vi "GUI_Pico_DMPicos.vi"() -> ()   [LabVIEW 2020]
uses:
  Shared/GUI_Template/GUI_master/tcp_new_data_event.ctl
  Shared/GUI_Template/GUI_master/tcp new data cluster.ctl
panel:
  in  "Position.device 1::2":dbl caption="Position X" min=-10000.0 max=10000.0
  in  "relativeMove.device 5neg::2":bool
  in  "relativeMove.device 5pos::2":bool
  in  "relativeMove.device 4neg::2":bool
  in  "relativeMove.device 4pos::2":bool
  in  "StepSize.device 5::2":dbl caption="StepSize Channel 5" min=0.0 max=1000.0
  in  "StepSize.device 4::2":dbl caption="StepSize Channel 4" min=0.0 max=1000.0
  in  "relativeMove.device 1neg::2":bool
  in  "relativeMove.device 1pos::2":bool
  in  "relativeMove.device 2pos::2":bool
  in  "relativeMove.device 2neg::2":bool
  in  "StepSize.device 2::2":dbl caption="StepSize Y-axis (2)" min=0.0 max=100.0
  in  "StepSize.device 1::2":dbl caption="StepSize X-axis (1)" min=0.0 max=100.0
  in  "GUIdevice 2":string="MCD-LT-PicoBooster"
  in  "stop":bool
  out "tcp data event":T1
  out "error IO 2":errorcluster
  # "XPW Input"
  # "PreAmp Input"
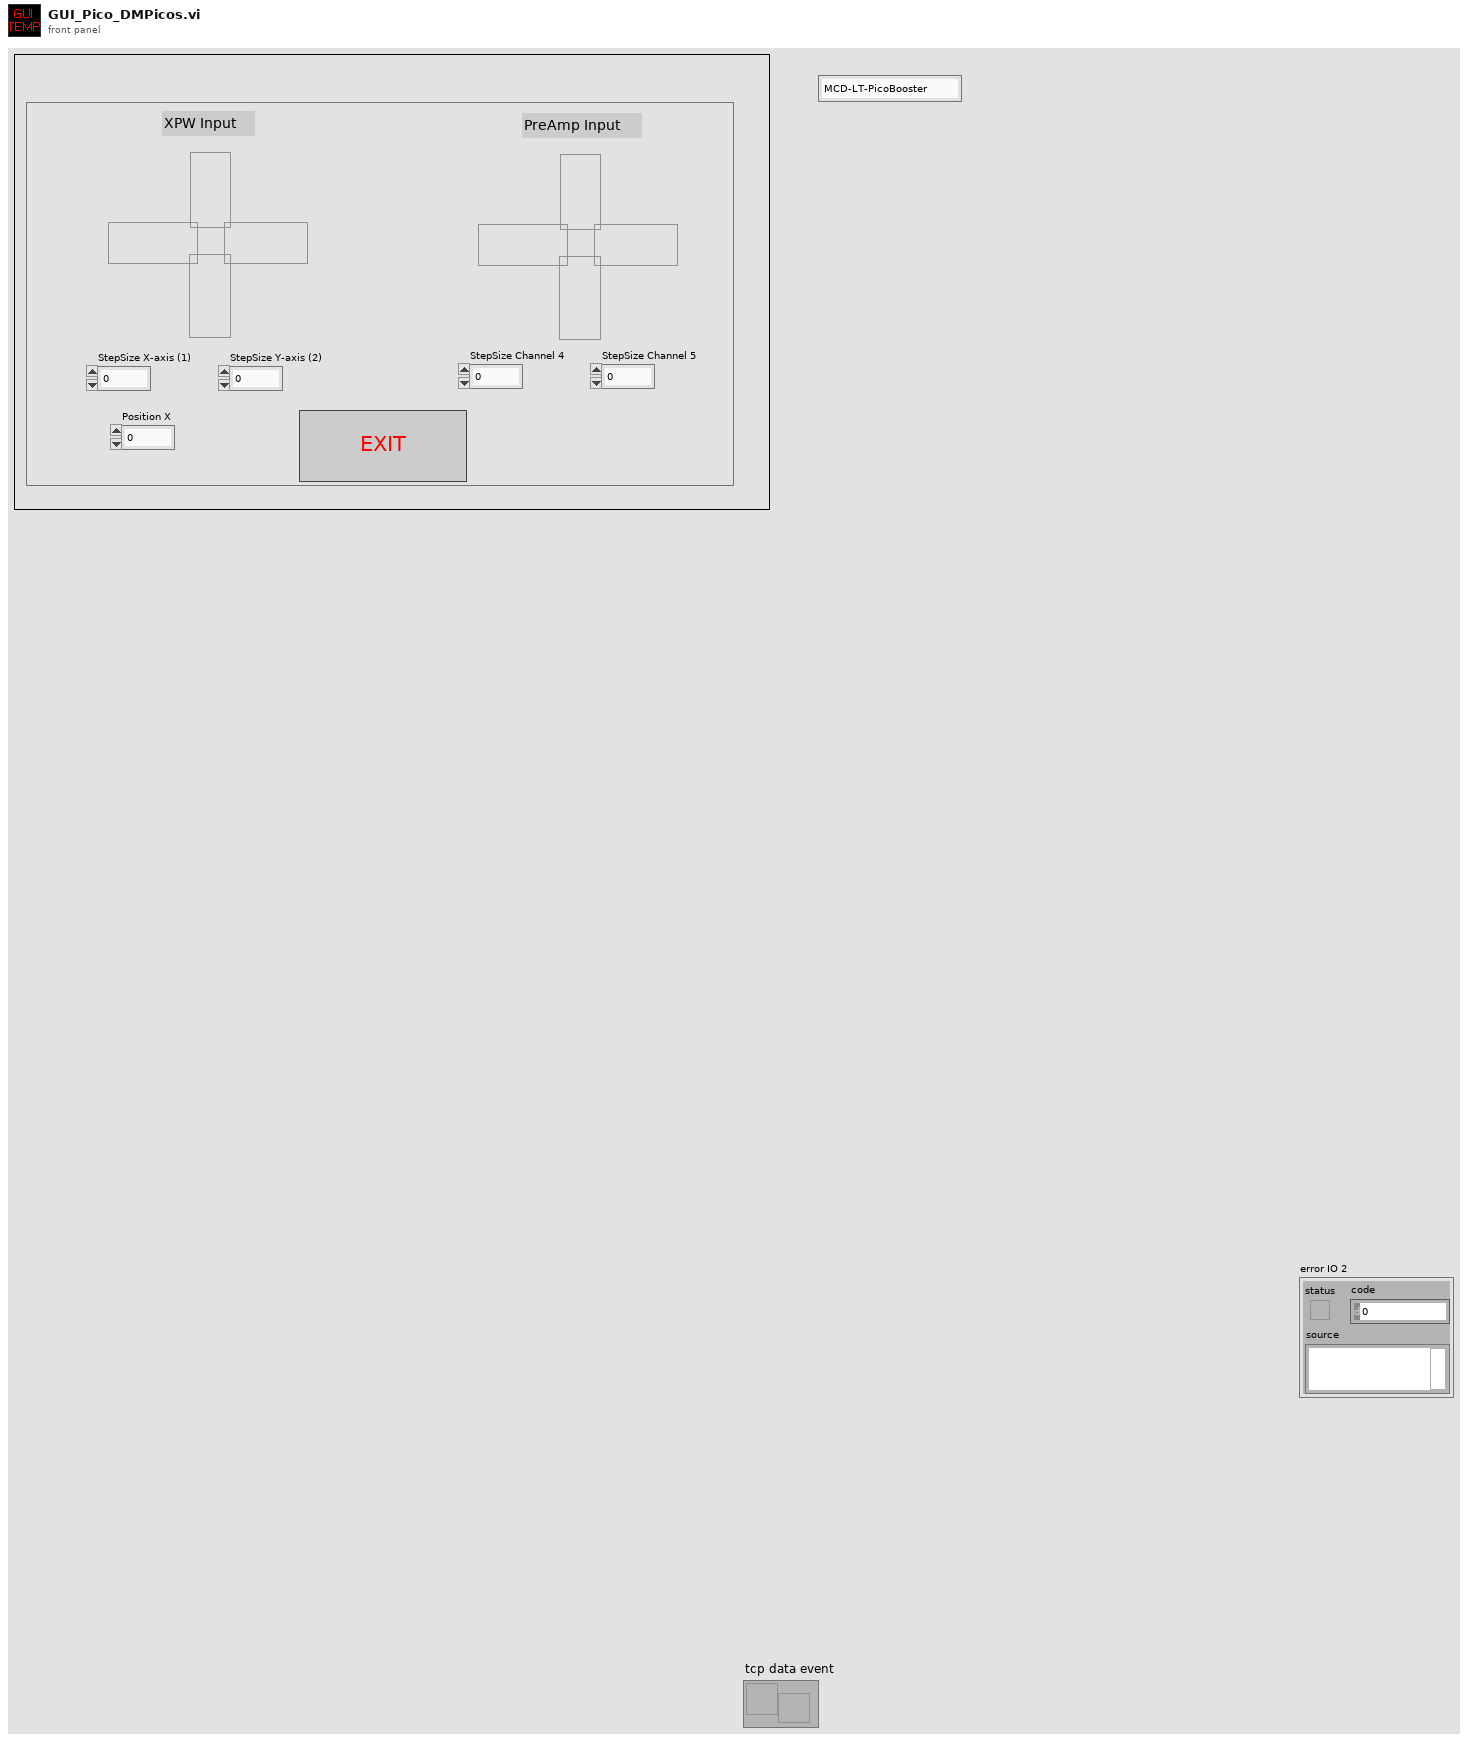
[diagram p1: front panel]
types:
  T1 = typedef "tcp_new_data_event.ctl" = refnum<user-event>
  T2 = typedef "tcp new data cluster.ctl" = cluster{"EventEnum":enum16{"new data", "connection status update"}, "Device name":string}
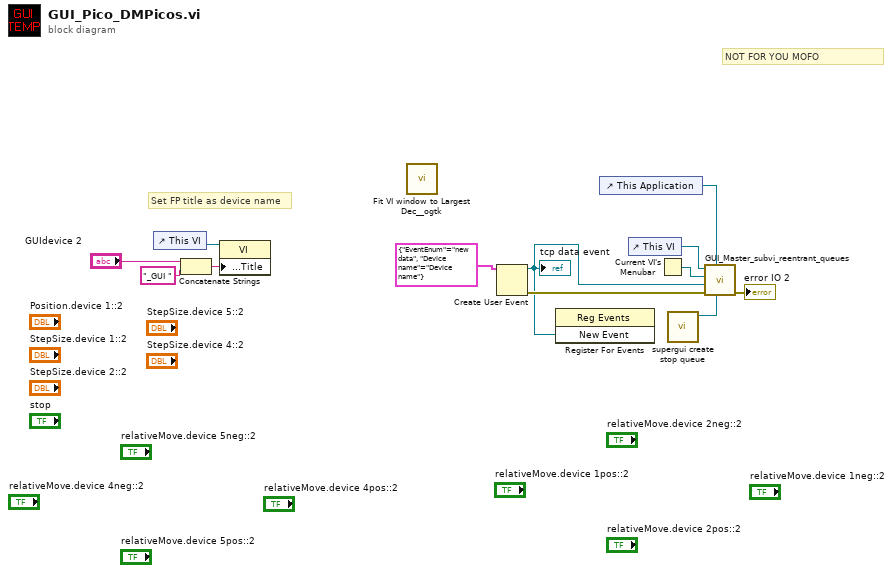
[diagram p0: block diagram]
diagram:
  # "Set FP title as device name"
  # "NOT FOR YOU MOFO"
  n1 = control-ref of="This VI"() -> (w4:refnum<vi>)
  n2 = Concatenate Strings("GUIdevice 2", "_GUI ") -> (w3:string)
  n3 = property class="VI"(reference=w4, "Front Panel.Title"=w3) -> ()  [unwired: 1 in, 2 out]
  n4 = call <userlib>:"Fit VI window to Largest Dec__ogtk.vi"() -> ()  [unwired: 6 in, 2 out]
  n5 = Create User Event(user event datatype=T2 {"EventEnum"=enum."new data", "Device name"="Device name"} ("New Event")) -> (user event=w7:refnum<user-event>, error out=w8:errorcluster)  [unwired: 1 in]
  "tcp data event" <- w7
  n6 = register-events(w7) -> ()  [unwired: 2 in, 2 out]
  n7 = control-ref of="This Application"() -> (w6:refnum<vi>)
  n8 = control-ref of="This VI"() -> (w11:refnum<vi>)
  n9 = Current VI's Menubar() -> (w10:refnum<k9>)
  n10 = call "supergui create stop queue.vi"() -> ("STOP Queue out"=w5:refnum<queue>)  [unwired: 11 in]
  n11 = call "GUI_Master_subvi_reentrant_queues.vi"("STOP Queue in"=w5, "This Application"=w6, "error in (no error)"=w8, "tcp data event"=w7, "Caller menu reference"=w10, "Caller VI ref"=w11) -> ("error out"=→"error IO 2":errorcluster)  [unwired: 5 in]
